vi "AutoCAD NET cmds by line.vi"(6 "AutoCAD cmd":T3, 8 "error in (no error)":errorcluster, 9 "Waveform Chart":refnum<vi>, 10 "Mathcad Output":T2, 11 "DesignRequest":T1) -> (0 "error out":errorcluster, 1 "Execution Time":dbl[](array[numeric]), 3 "DesignRequest out":T1)   [LabVIEW 2011]
uses:
  AutoCAD cmds.ctl
  Design Request.ctl
  Variable cluster.ctl
  Autodesk.AutoCAD.Interop
  Design Server.lvlib
panel:
  out "milliseconds":dbl
  out "Version":string
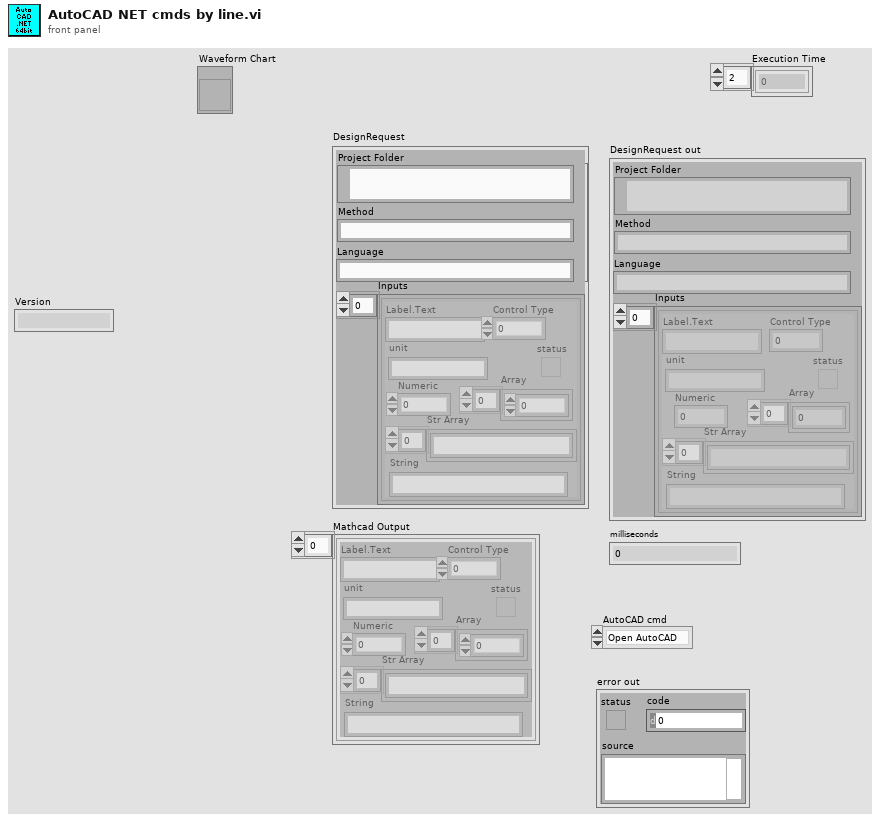
[diagram p1: front panel]
types:
  T1 = typedef "Design Server.lvlib/Design Request.ctl" = cluster{"Project Folder":path, "Method":string, "Inputs":T2, "Language":string}
  T2 = typedef "Design Server.lvlib/Variable cluster.ctl" = cluster{"Label.Text":string, "Control Type":u32, "Numeric":dbl, "Array":dbl[], "status":bool, "Str Array":string[], "String":string, "unit":string}[]
  T3 = typedef "Design Server.lvlib/AutoCAD cmds.ctl" = enum16{"Open AutoCAD", "Create Drawing", "Quit"}
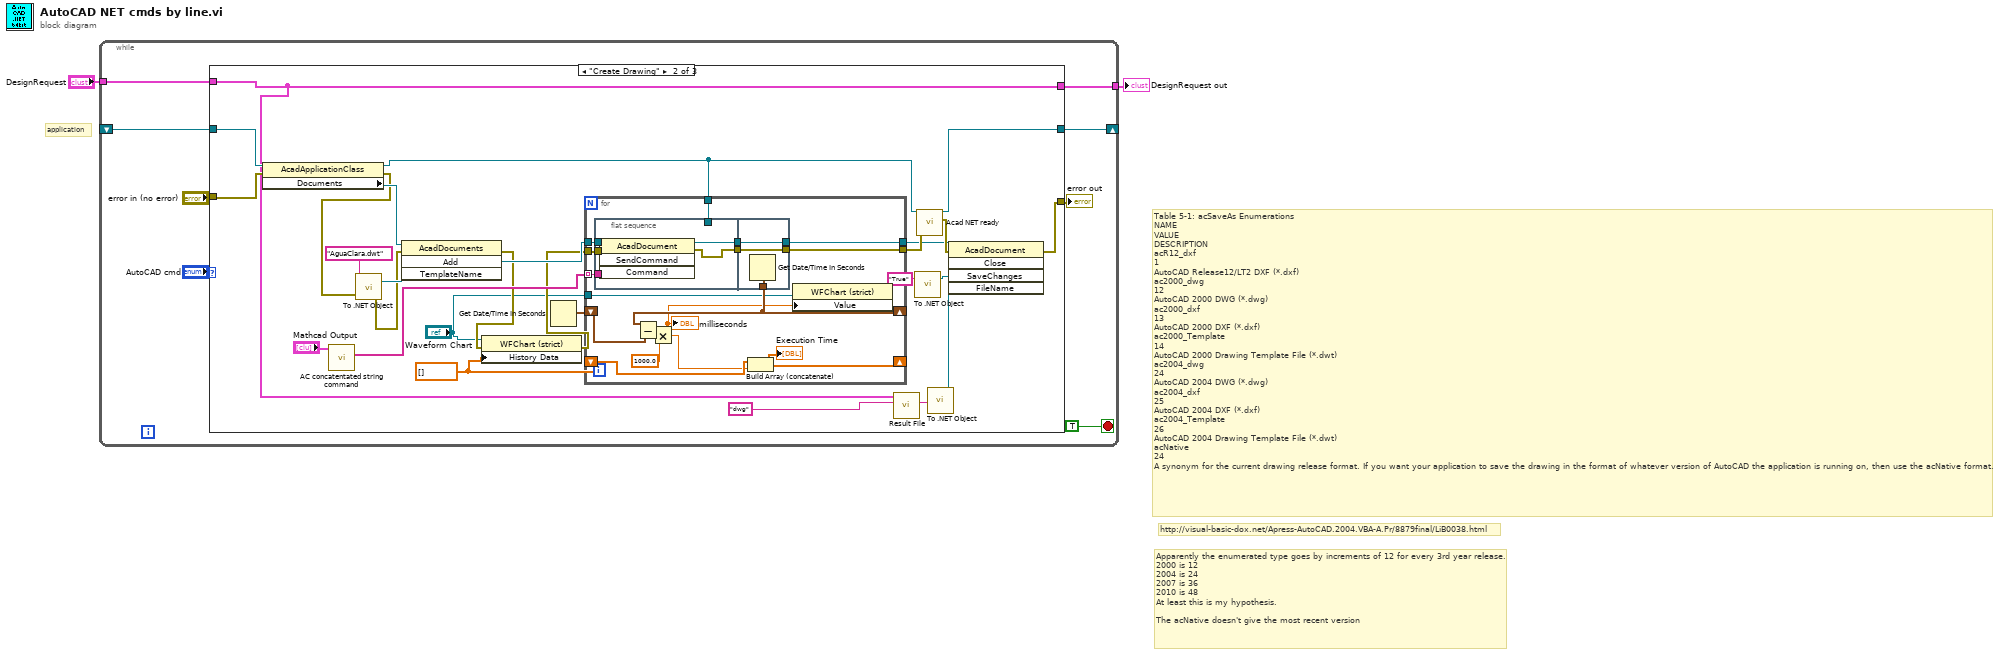
[diagram p0: block diagram]
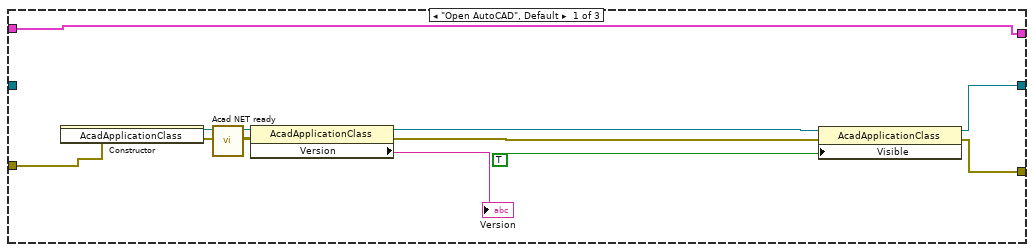
[diagram p2: hidden frame]
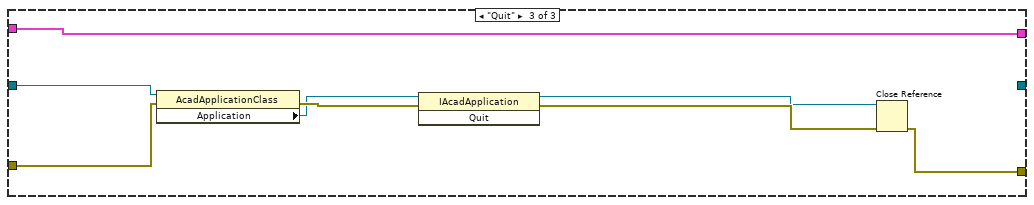
[diagram p3: hidden frame]
diagram:
  # "Apparently the enumerated type goes by increments of 12 for every 3rd year release.\n2000 is 12\n2004 is 24\n2007 is 36\n2010 is 48\nAt least this is my hypothesis. \n\nThe acNative doesn't give the most recent version"
  # "http://visual-basic-dox.net/Apress-AutoCAD.2004.VBA-A.Pr/8879final/LiB0038.html"
  # "Table 5-1: acSaveAs Enumerations\nNAME\nVALUE\nDESCRIPTION\nacR12_dxf\n1\nAutoCAD Release12/LT2 DXF (*.dxf)\nac2000_dwg\n12\nAutoCAD 2000 DWG (*.dwg)\nac2000_dxf\n13\nAutoCAD 2000 DXF (*.dxf)\nac2000_Template\n14\nAutoCAD 2000 Drawing Template File (*.dwt)\nac2004_dwg\n24\nAutoCAD 2004 DWG (*.dwg)\nac2004_dxf\n25\nAutoCAD 2004 DXF (*.dxf)\nac2004_Template\n26\nAutoCAD 2004 Drawing Template File (*.dwt)\nacNative\n24\nA synonym for the current drawing release format. If you want your application to save the drawing in the format of whatever version of AutoCAD the application is running on, then use the acNative format."
  # "application"
  n1 = while {
    shift-right: [w9] -> _
    shift-left: _ -> [w6]
    tunnel: [w4] -> w2
    tunnel: "DesignRequest" -> [w3]
    stop <- TRUE stop-if-true
    n2 = case shown="\"Create Drawing\"" "AutoCAD cmd" {
      tunnel: [w12 w31 _] -> w9
      tunnel: "error in (no error)" -> [w16 w49 w76]
      tunnel: [w11 w38 w75] -> w7
      tunnel: w6 -> [_ w48 w77]
      tunnel: [w22 w36 w81] -> w4
      tunnel: w3 -> [w22 w36 w81]
      frame "Open AutoCAD", Default {
        n3 = constructor class="AcadApplicationClass"(error in=w16) -> (reference out=w20:refnum<k24>, error out=w18:errorcluster)  [unwired: 2 in, 1 out]
        n4 = call "Acad NET ready.vi"("error in (no error)"=w18, ".NET Refnum in"=w20) -> ("error out"=w17:errorcluster, "reference out"=w19:refnum<k24>)  [unwired: 8 in]
        n5 = property class="AcadApplicationClass"(reference=w19, error in=w17) -> (reference out=w13:refnum<k24>, error out=w14:errorcluster, "Version"=→"Version":string)
        n6 = property class="AcadApplicationClass"(reference=w13, error in=w14, "Visible"=TRUE) -> (reference out=w12:refnum<k24>, error out=w11:errorcluster)
      }
      frame "Create Drawing" {
        w25 = dbl[] []
        n7 = property class="AcadApplicationClass"(reference=w48, error in=w49) -> (reference out=w23:refnum<k24>, error out=w40:errorcluster, "Documents"=w41:refnum<k24>)
        n8 = call "AC concatentated string command.vi"("MathCAD results"="Mathcad Output") -> ("AC array"=w29:string[])  [unwired: 9 in, 1 out]
        n9 = call <vilib>:"To .NET Object.vi"("error in (no error)"=w40, "anything"="AguaClara.dwt") -> ("error out"=w39:errorcluster, ".NET object"=w46:refnum<k24>)
        n10 = invoke class="AcadDocuments" method="Add"(reference=w41, error in=w39, "TemplateName"=w46) -> (error out=w27:errorcluster, "Add"=w47:refnum<k24>)  [unwired: 1 in, 2 out]
        n11 = property class="WFChart (strict)"(reference="Waveform Chart", error in=w27, "History Data"=w25) -> (error out=w26:errorcluster)  [unwired: 1 out]
        n12 = Get Date/Time In Seconds() -> (seconds since 1Jan1904=w28:timestamp)
        n13 = for {
          tunnel: w26 -> [w65]
          tunnel: w47 -> [w64]
          tunnel: [w63] -> w33
          tunnel: [w62] -> w30
          tunnel: w29 -> [w61] mode=indexing
          shift-right: [w55] -> _
          shift-left: w28 -> [w58]
          shift-right: [w53] -> _
          shift-left: w25 -> [w54]
          tunnel: "Waveform Chart" -> [w52]
          tunnel: w23 -> [w50]
          n14 = flat-sequence {
            tunnel: w65 -> [w70]
            tunnel: w64 -> [w69]
            tunnel: w61 -> [w68]
            tunnel: [w66] -> w57
            tunnel: [w67] -> w56
            tunnel: w50 -> [_]
            tunnel: [w72] -> w62
            tunnel: [w73] -> w63
            tunnel: w57 -> [w73]
            tunnel: w56 -> [w72]
            tunnel: [w71] -> w55
            frame #0 {
              n15 = invoke class="AcadDocument" method="SendCommand"(reference=w69, error in=w70, "Command"=w68) -> (reference out=w67:refnum<k24>, error out=w66:errorcluster)  [unwired: 1 in, 2 out]
            }
            frame #1 {
              n16 = Get Date/Time In Seconds() -> (seconds since 1Jan1904=w71:timestamp)
            }
          }
          n17 = Subtract(x=w55, y=w58) -> (x-y=w60:dbl)
          n18 = Multiply(x=w60, y=1000.0) -> (x*y=w51:dbl)
          "milliseconds" <- w51
          n19 = Build Array (concatenate)(w54, w51) -> (w53:dbl[])
          "Execution Time" <- w53
          n20 = property class="WFChart (strict)"(reference=w52, "Value"=w51) -> ()  [unwired: 1 in, 2 out]
        }
        n21 = call "Result File.vi"("File Type"="dwg", "DesignRequest"=w36) -> ("File string"=w37:string)  [unwired: 8 in, 1 out]
        n22 = call <vilib>:"To .NET Object.vi"("anything"="True") -> (".NET object"=w44:refnum<k24>)  [unwired: 1 in, 1 out]
        n23 = call "Acad NET ready.vi"("error in (no error)"=w33, ".NET Refnum in"=w23) -> ("error out"=w32:errorcluster, "reference out"=w31:refnum<k24>)  [unwired: 8 in]
        n24 = call <vilib>:"To .NET Object.vi"("anything"=w37) -> (".NET object"=w45:refnum<k24>)  [unwired: 1 in, 1 out]
        n25 = invoke class="AcadDocument" method="Close"(reference=w30, error in=w32, "SaveChanges"=w44, "FileName"=w45) -> (error out=w38:errorcluster)  [unwired: 1 in, 4 out]
      }
      frame "Quit" {
        n26 = property class="AcadApplicationClass"(reference=w77, error in=w76) -> (error out=w80:errorcluster, "Application"=w79:refnum<k24>)  [unwired: 1 out]
        n27 = invoke class="IAcadApplication" method="Quit"(reference=w79, error in=w80) -> (reference out=w74:refnum<k24>, error out=w78:errorcluster)  [unwired: 1 in, 1 out]
        n28 = Close Reference(reference=w74, error in (no error)=w78) -> (error out=w75:errorcluster)
      }
    }
    "error out" <- w7
  }
  "DesignRequest out" <- w2
